vi "Shared_DCPower_Start.vi"(7 "DCPowerParameters":T1[](array[typedef]) {"Source Delay" format="%.6p"; "Sense" items=["Local"=1008, "Remote"=1009]; "Aperture_time" format="%.6p"; "Current_range" format="%.6p"; "Current" format="%.6p"; "Voltage_range" format="%.6p"; "Voltage" format="%.6p"}, 10 "Pins":tag[](array[tag]), 11 "Semiconductor Module Context":T2) -> (0 "error Out":errorcluster)   [LabVIEW 2023, in "Shared.lvlib"]
doc: "Start supplying Voltage on the System Power Supply for Relay control"
uses:
  Shared.lvlib
  <vilib>/NI_TestStand_SemiconductorModule/NI_TestStand_Semiconductor_Module.lvlibp/PinMap/General/SemiconductorModuleContext.ctl
  ResourceHandling/TypeDefs/RH_DCPower_Parameters.ctl
  <vilib>/NI_TestStand_SemiconductorModule/NI_TestStand_Semiconductor_Module.lvlibp/PinMap/DC Power/PinsToNIDCPowerSessions.vi
  <vilib>/NI_TestStand_SemiconductorModule/NI_TestStand_Semiconductor_Module.lvlibp
  ResourceHandling/ResourceHandling.lvlib
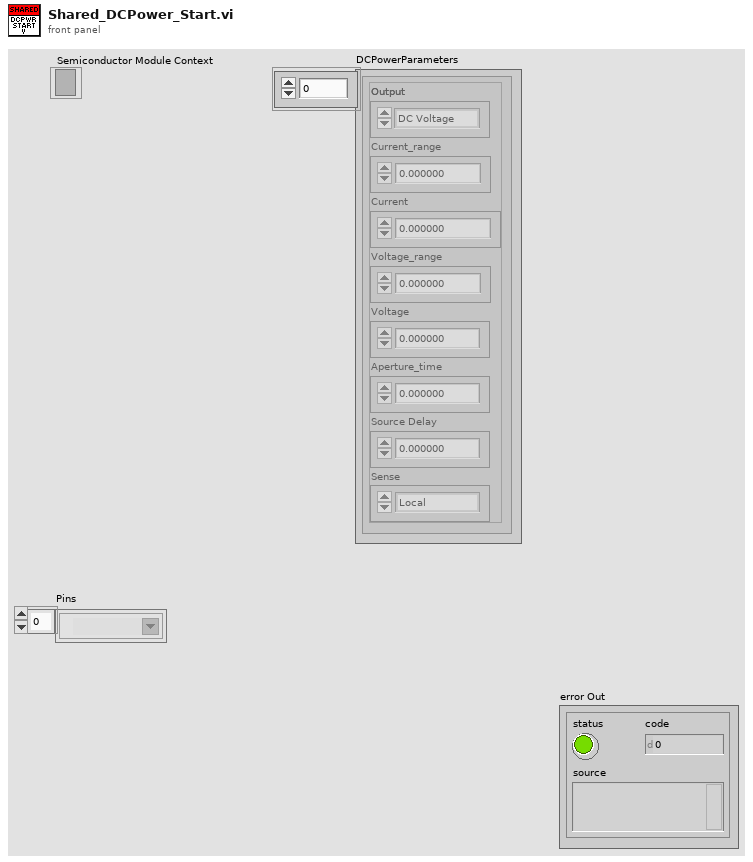
[diagram p1: front panel]
types:
  T1 = typedef "ResourceHandling.lvlib/RH_DCPower_Parameters.ctl" = cluster{"Output":enum16{"DC Voltage", "DC Current"}, "Current_range":dbl, "Current":dbl, "Voltage_range":dbl, "Voltage":dbl, "Aperture_time":dbl, "Source Delay":dbl, "Sense":i32}
  T2 = typedef "NI_TestStand_Semiconductor_Module.lvlibp/SemiconductorModuleContext.ctl" = refnum<k7>
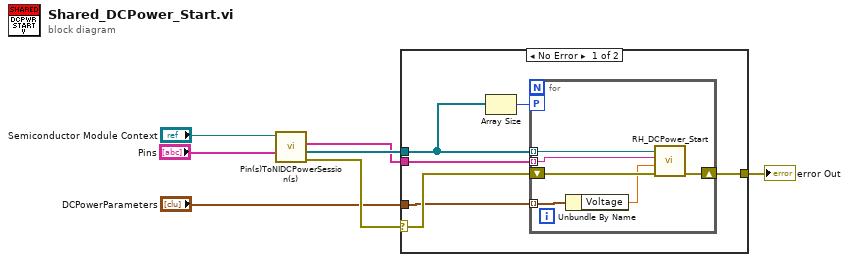
[diagram p0: block diagram]
diagram:
  n1 = call-poly <vilib>:"Pin(s)ToNIDCPowerSession(s).vi"("Pins"="Pins", "Semiconductor Module Context"="Semiconductor Module Context") -> ("error out"=w6:errorcluster, "Instrument Sessions"=w5:refnum<k15>[], "Channel Strings"=w4:string[])  [unwired: 5 in, 2 out]
  n2 = case shown="No Error" w6 {
    selector: w6 -> [w9 w20]
    tunnel: w5 -> [w12 _]
    tunnel: w4 -> [w11 _]
    tunnel: [w10 w20] -> w3
    tunnel: "DCPowerParameters" -> [w8 _]
    frame No Error {
      n3 = Array Size(array=w12) -> (size(s)=w13:i32)
      n4 = for {
        tunnel: w12 -> [w19] mode=indexing
        workers-P: w13 -> [_]
        tunnel: w11 -> [w18] mode=indexing
        shift-right: [w17] -> w10
        shift-left: w9 -> [w16]
        tunnel: w8 -> [w15] mode=indexing
        n5 = Unbundle By Name(w15) -> ("Voltage"=w14:dbl)
        n6 = call "RH_DCPower_Start.vi"("error in (no error)"=w16, "Voltage"=w14, "Channel List"=w18, "DCPower Session In"=w19) -> ("error out"=w17:errorcluster)  [unwired: 6 in, 1 out]
      }
    }
    frame Error {
    }
  }
  "error Out" <- w3
